vi "remove all keys from a sector.vi"(7 "sector":string, 8 "error in (no error)":errorcluster, 11 "file name":string) -> (0 "error out":errorcluster)   [LabVIEW 2024]
uses:
  <vilib>/Utility/config.llb/NI_LVConfig.lvlib
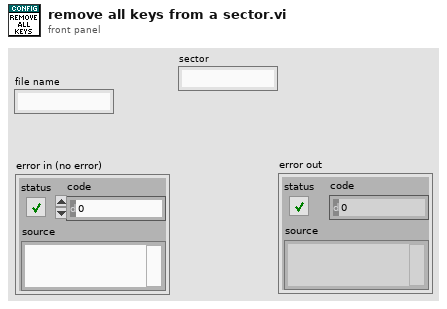
[diagram p1: front panel]
types:
  T1 = typedef "NI_LVConfig.lvlib/Config Data RefNum.ctl" = refnum<k1>
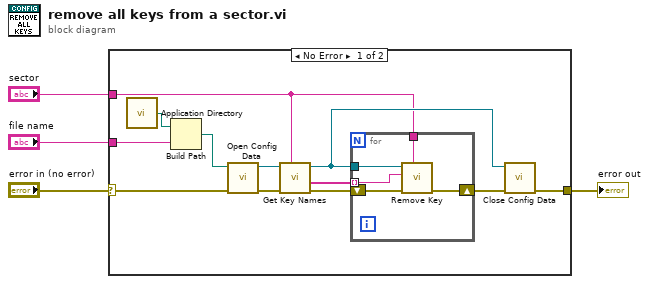
[diagram p0: block diagram]
diagram:
  n1 = case shown="No Error" "error in (no error)" {
    selector: "error in (no error)" -> [w5 w22]
    tunnel: [w16 w22] -> w4
    tunnel: "sector" -> [w11 _]
    tunnel: "file name" -> [w8 _]
    frame No Error {
      n2 = call <vilib>:"Application Directory.vi"() -> ("Application Directory"=w7:path)
      n3 = Build Path(base path=w7, name or relative path=w8) -> (appended path=w6:path)
      n4 = call <vilib>:"Open Config Data.vi"("error in (no error)"=w5, "configuration file path"=w6) -> ("error out"=w9:errorcluster, "refnum"=w10:T1)  [unwired: 7 in, 1 out]
      n5 = call <vilib>:"Get Key Names.vi"("section"=w11, "error in (no error)"=w9, "refnum"=w10) -> ("error out"=w12:errorcluster, "key names"=w13:string[], "refnum out"=w15:T1)  [unwired: 5 in, 1 out]
      n6 = for {
        tunnel: w11 -> [w21]
        tunnel: w15 -> [w19]
        tunnel: w13 -> [w18] mode=indexing
        shift-right: [w17] -> w14
        shift-left: w12 -> [w20]
        n7 = call <vilib>:"Remove Key.vi"("section"=w21, "error in (no error)"=w20, "key"=w18, "refnum"=w19) -> ("error out"=w17:errorcluster)  [unwired: 5 in, 2 out]
      }
      n8 = call <vilib>:"Close Config Data.vi"("error in (no error)"=w14, "refnum"=w15) -> ("error out"=w16:errorcluster)  [unwired: 8 in, 1 out]
    }
    frame Error {
    }
  }
  "error out" <- w4
